vi "update and log odors LabJack.vi"(7 "global enable":bool, 8 "error in":errorcluster, 9 "t0":u32, 10 "gradient settings":T5={"background air settings"={"enabled"=FALSE, "temporal ramp type"=enum."Sine", "period(s)"=120.0, "high limit"=100.0, "low limit"=0.0, "duty cycle (sq wave)"=50.0, "phase shift (deg)"=0.0, "value to output when disabled"=0.0}, "odor1 settings"={"enabled"=FALSE, "temporal ramp type"=enum."Sine", "period(s)"=120.0, "high limit"=100.0, "low limit"=0.0, "duty cycle (sq wave)"=50.0, "phase shift (deg)"=0.0, "value to output when disabled"=0.0}, "dilution air"={"enabled"=FALSE, "temporal ramp type"=enum."Sine", "period(s)"=120.0, "high limit"=100.0, "low limit"=0.0, "duty cycle (sq wave)"=50.0, "phase shift (deg)"=0.0, "value to output when disabled"=0.0}} {"dilution air"."value to output when disabled" max=100.0; "dilution air"."low limit" min=0.0 max=1.0 format="%#_6p"; "dilution air"."high limit" max=100.0; "odor1 settings"."value to output when disabled" max=100.0; "odor1 settings"."low limit" min=0.0 max=1.0 format="%#_6p"; "odor1 settings"."high limit" max=100.0; "background air settings"."value to output when disabled" max=100.0; "background air settings"."low limit" min=0.0 max=1.0 format="%#_6p"; "background air settings"."high limit" max=100.0}, 11 "LabJack Tasks":T2) -> (0 "error out":errorcluster, 2 "flow rates":T3 {"pid reading" format="%0.2f"}, 3 "setpoints":T4)   [LabVIEW 2021]
uses:
  LabJack Interface/LabJack AOAI Channel.ctl
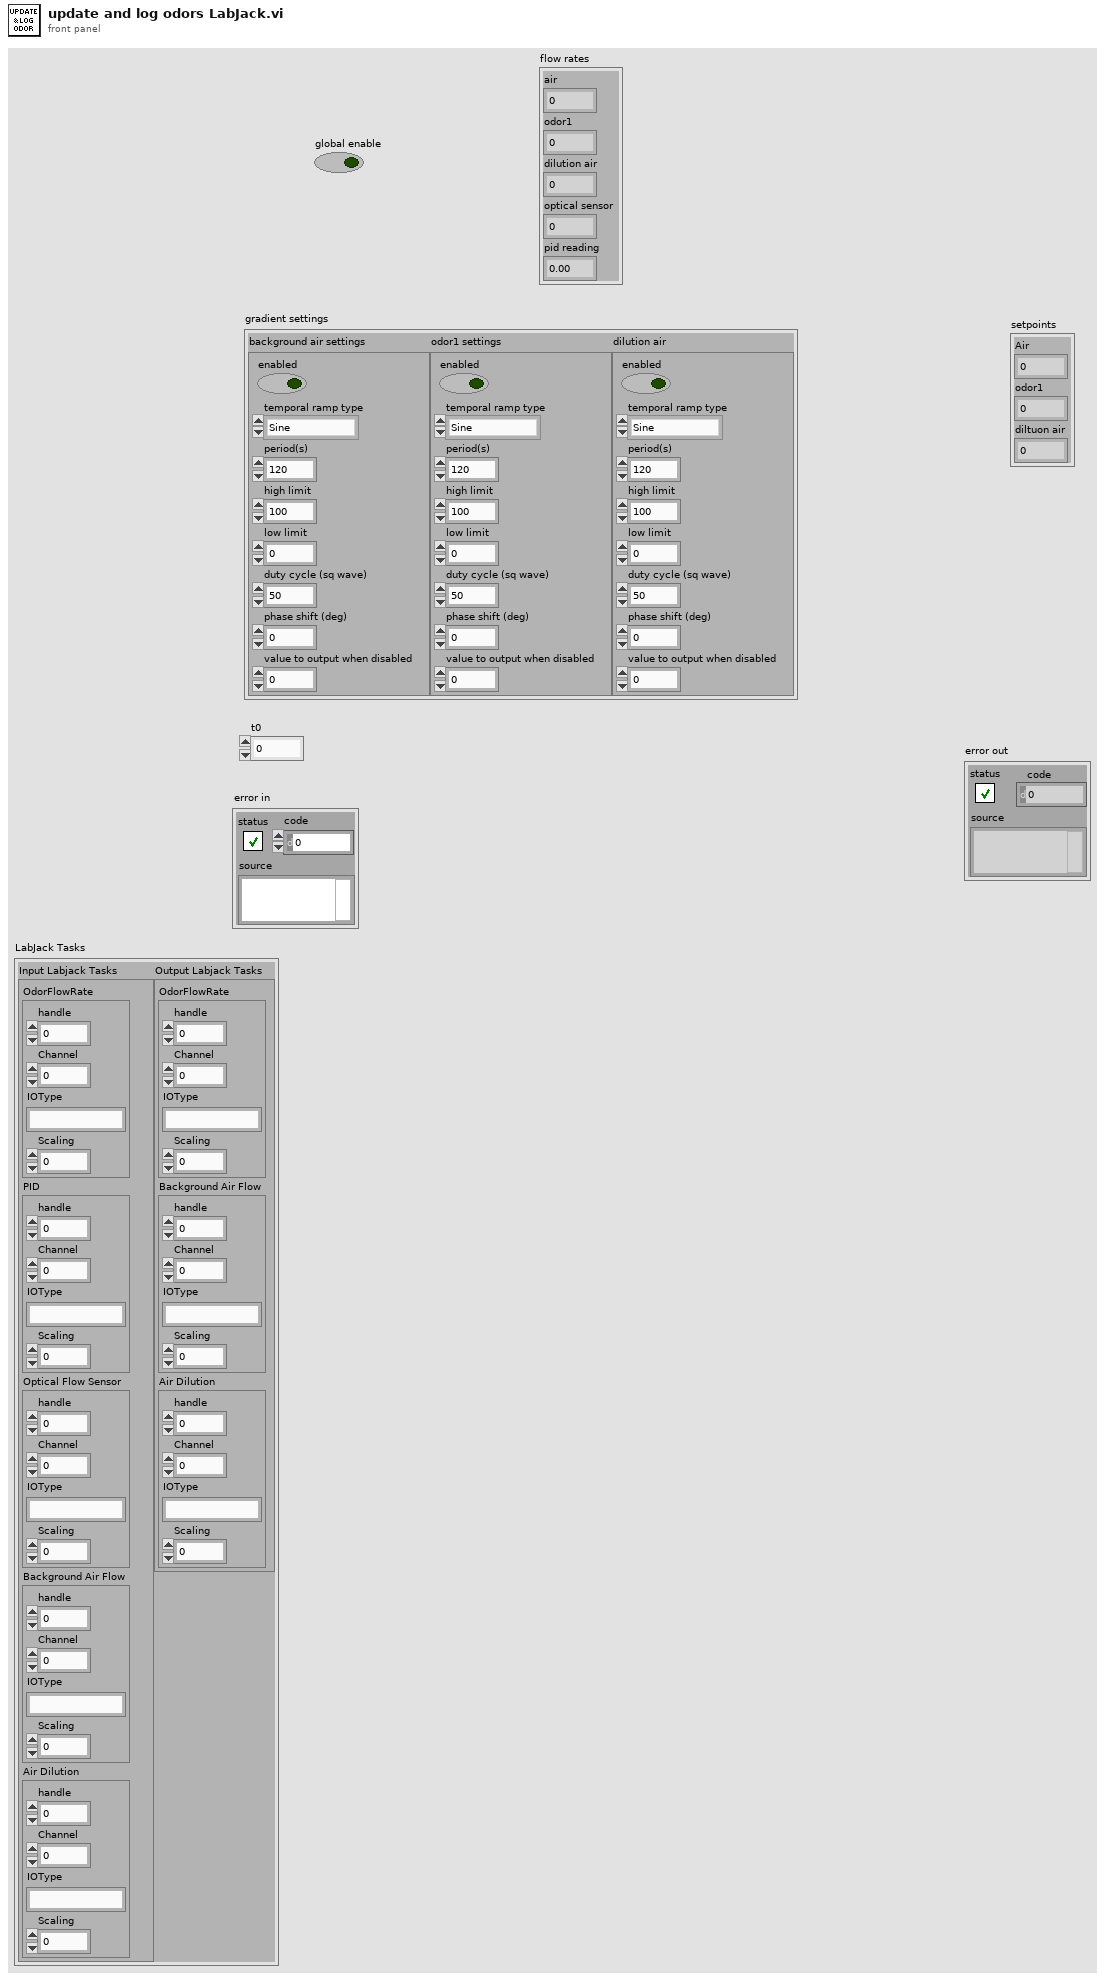
[diagram p1: front panel]
types:
  T1 = typedef "LabJack AOAI Channel.ctl" = cluster{"handle":i32, "Channel":i32, "IOType":string, "Scaling":dbl}
  T2 = cluster{"Input Labjack Tasks":cluster{"OdorFlowRate":T1, "PID":T1, "Optical Flow Sensor":T1, "Background Air Flow":T1, "Air Dilution":T1}, "Output Labjack Tasks":cluster{"OdorFlowRate":T1, "Background Air Flow":T1, "Air Dilution":T1}}
  T3 = cluster{"air":dbl, "odor1":dbl, "dilution air":dbl, "optical sensor":dbl, "pid reading":dbl}
  T4 = cluster{"Air ":dbl, "odor1":dbl, "diltuon air":dbl}
  T5 = cluster{"background air settings":cluster{"enabled":bool, "temporal ramp type":enum16{"Sine", "Triangle", "Sawtooth", "Square", "Exponential"}, "period(s)":dbl, "high limit":dbl, "low limit":dbl, "duty cycle (sq wave)":dbl, "phase shift (deg)":dbl, "value to output when disabled":dbl}, "odor1 settings":cluster{"enabled":bool, "temporal ramp type":enum16{"Sine", "Triangle", "Sawtooth", "Square", "Exponential"}, "period(s)":dbl, "high limit":dbl, "low limit":dbl, "duty cycle (sq wave)":dbl, "phase shift (deg)":dbl, "value to output when disabled":dbl}, "dilution air":cluster{"enabled":bool, "temporal ramp type":enum16{"Sine", "Triangle", "Sawtooth", "Square", "Exponential"}, "period(s)":dbl, "high limit":dbl, "low limit":dbl, "duty cycle (sq wave)":dbl, "phase shift (deg)":dbl, "value to output when disabled":dbl}}
  T6 = cluster{"enabled":bool, "temporal ramp type":enum16{"Sine", "Triangle", "Sawtooth", "Square", "Exponential"}, "period(s)":dbl, "high limit":dbl, "low limit":dbl, "duty cycle (sq wave)":dbl, "phase shift (deg)":dbl, "value to output when disabled":dbl}[]
  T7 = enum16{"Sine", "Triangle", "Sawtooth", "Square", "Exponential"}
  T8 = cluster{"temporal ramp type":enum16{"Sine", "Triangle", "Sawtooth", "Square", "Exponential"}, "period(s)":dbl, "high limit":dbl, "low limit":dbl, "duty cycle (sq wave)":dbl, "phase shift (deg)":dbl, "value to output when disabled":dbl}
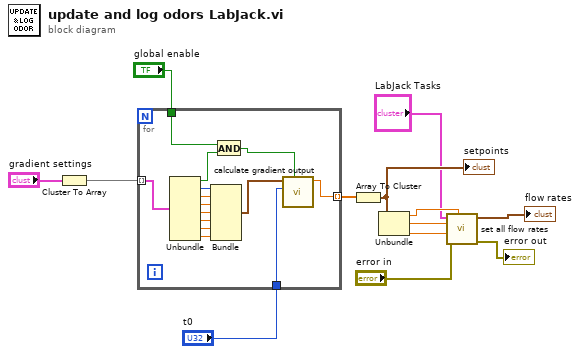
[diagram p0: block diagram]
diagram:
  n1 = Cluster To Array(cluster="gradient settings") -> (array=w12:T6)
  n2 = for {
    tunnel: w12 -> [w27] mode=indexing
    tunnel: "t0" -> [w18]
    tunnel: "global enable" -> [w16]
    tunnel: [w14] -> w9 mode=indexing
    n3 = Unbundle(w27) -> ("enabled"=w17:bool, "temporal ramp type"=w26:T7, "period(s)"=w20:dbl, "high limit"=w21:dbl, "low limit"=w22:dbl, "duty cycle (sq wave)"=w23:dbl, "phase shift (deg)"=w24:dbl, "value to output when disabled"=w25:dbl)
    n4 = Bundle("temporal ramp type"=w26, "period(s)"=w20, "high limit"=w21, "low limit"=w22, "duty cycle (sq wave)"=w23, "phase shift (deg)"=w24, "value to output when disabled"=w25) -> (w19:T8)  [unwired: 1 in]
    n5 = And(x=w16, y=w17) -> (x .and. y?=w15:bool)
    n6 = call "calculate gradient output.vi"("enabled"=w15, "t0"=w18, "gradient parameters"=w19) -> ("value out"=w14:dbl)  [unwired: 8 in]
  }
  n7 = Array To Cluster(array=w9) -> (cluster=w8:cluster{"[0]":dbl, "[1]":dbl, "[2]":dbl})
  "setpoints" <- w8
  n8 = Unbundle(w8) -> ("[0]"=w7:dbl, "[1]"=w6:dbl, "[2]"=w5:dbl)
  n9 = call "set all flow rates.vi"("background air flow rate"=w7, "error in"="error in", "dilution air flow rate"=w5, "odor 1 flow rate"=w6, "LabJack Tasks"="LabJack Tasks") -> ("error out"=→"error out":errorcluster, "flow rates"=→"flow rates":T3)  [unwired: 5 in]
